vi "setup.vi"   [LabVIEW 2015]
uses:
  phlib.dll
types:
  T1 = cluster{"initialized":bool, "devidx":i32, "Ch0 Level":i32, "Ch0 ZeroX":i32, "Ch1 Level":i32, "Ch1 ZeroX":i32, "sync rate":i32, "resolution":i32, "acq time":i32, "acq rate":i32, "# bins":u32, "Bin size":enum16{"1", "2", "4", "8", "16", "32", "64", "128"}, "min photons":u32, "truncate":u32}
  T2 = enum16{"1", "2", "4", "8", "16", "32", "64", "128"}
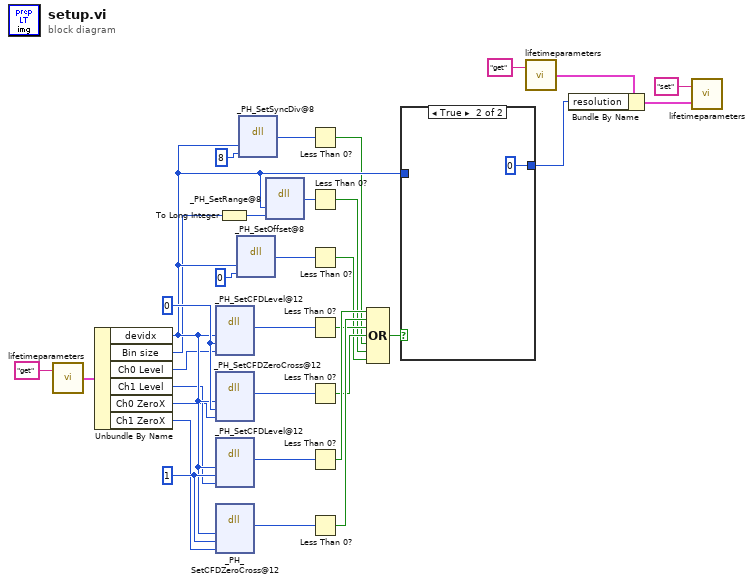
[diagram p0: block diagram]
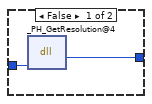
[diagram p2: hidden frame]
diagram:
  w25 = 0
  w26 = 1
  n1 = call "lifetimeparameters.vi"("command"="get") -> ("Params out"=w23:T1)  [unwired: 1 in]
  n2 = Unbundle By Name(w23) -> ("devidx"=w22:i32, "Bin size"=w12:T2, "Ch0 Level"=w6:i32, "Ch1 Level"=w9:i32, "Ch0 ZeroX"=w7:i32, "Ch1 ZeroX"=w8:i32)
  n3 = dll-call lib="phlib.dll" fn="_PH_SetCFDLevel@12"("devidx"=w22, "channel"=w25, "Level"=w6) -> (w29:i32)  [unwired: 6 in, 2 out]
  n4 = dll-call lib="phlib.dll" fn="_PH_SetCFDZeroCross@12"("devidx"=w22, "channel"=w25, "Level"=w7) -> (w28:i32)  [unwired: 6 in, 2 out]
  n5 = dll-call lib="phlib.dll" fn="_PH_SetCFDLevel@12"("devidx"=w22, "channel"=w26, "Level"=w9) -> (w33:i32)  [unwired: 6 in, 2 out]
  n6 = dll-call lib="phlib.dll" fn="_PH_SetCFDZeroCross@12"("devidx"=w22, "channel"=w26, "Level"=w8) -> (w30:i32)  [unwired: 6 in, 2 out]
  n7 = To Long Integer(number=w12) -> (32bit integer=w11:i32)
  n8 = dll-call lib="phlib.dll" fn="_PH_SetOffset@8"("devidx"=w22, "Offset"=0) -> (w31:i32)  [unwired: 5 in, 2 out]
  n9 = dll-call lib="phlib.dll" fn="_PH_SetSyncDiv@8"("devidx"=w22, "divider"=8) -> (w27:i32)  [unwired: 5 in, 2 out]
  n10 = dll-call lib="phlib.dll" fn="_PH_SetRange@8"("devidx"=w22, "Range"=w11) -> (w32:i32)  [unwired: 5 in, 2 out]
  n11 = Less Than 0?(x=w27) -> (x < 0?=w15:bool)
  n12 = Less Than 0?(x=w32) -> (x < 0?=w14:bool)
  n13 = Less Than 0?(x=w31) -> (x < 0?=w13:bool)
  n14 = Less Than 0?(x=w29) -> (x < 0?=w17:bool)
  n15 = Less Than 0?(x=w28) -> (x < 0?=w16:bool)
  n16 = Less Than 0?(x=w33) -> (x < 0?=w19:bool)
  n17 = Less Than 0?(x=w30) -> (x < 0?=w18:bool)
  n18 = Compound Arithmetic op=OR(w19, w18, w17, w16, w15, w14, w13) -> (w20:bool)
  n19 = case shown="True" w20 {
    tunnel: [w35 0] -> w1
    tunnel: w22 -> [w34 _]
    frame False {
      n20 = dll-call lib="phlib.dll" fn="_PH_GetResolution@4" label="PH_GetResolution"("devidx"=w34) -> (w35:i32)  [unwired: 4 in, 2 out]
    }
    frame True {
    }
  }
  n21 = call "lifetimeparameters.vi"("command"="get") -> ("Params out"=w3:T1)  [unwired: 1 in]
  n22 = Bundle By Name(cluster=w3, "resolution"=w1) -> (w2:T1)
  n23 = call "lifetimeparameters.vi"("Params in"=w2, "command"="set") -> ()  [unwired: 1 out]
